vi "VisionGlobal.vi"() -> ()   [LabVIEW 2023]
uses:
  <vilib>/Rock Robotics/WPI/ThirdParty/JAS_Junk/TrajLib/TypeDef/POSE2D.ctl
  <vilib>/Rock Robotics/WPI/ThirdParty/JAS_Junk/TrajLib/TypeDef/TRANSLATION2D.ctl
  <vilib>/Rock Robotics/WPI/ThirdParty/JAS_Junk/TrajLib/TypeDef/ROTATION2D.ctl
  <vilib>/Rock Robotics/WPI/ThirdParty/JAS_Junk/TrajLib/Trajectory_Library.lvlib
panel:
  out "Vision_Right_HasTarg":bool
  out "Vision_Right_NewData":bool
  out "Vision_Left_HasTarg":bool
  out "Vision_Left_NewData":bool
  out "Vision_LeftTime_Sec":dbl
  out "Vision_RightAng_Deg":dbl
  out "Vision_RightY_Ft":dbl
  out "Vision_RightX_Ft":dbl
  out "Vision_RightTime_Sec":dbl
  out "Vision_LeftAng_Deg":dbl
  out "Vision_LeftY_Ft":dbl
  out "Vision_LeftX_Ft":dbl
  out "VisionFPGATime":dbl
  out "Vision Conn L":bool
  out "Vision Count L":dbl=-1.0
  out "Vision Err L":bool
  out "Vision Conn R":bool
  out "Vision Count R":dbl=-1.0
  out "Vision Err R":bool
  out "Odom Error":bool
  in  "Current ABS Pose":T1={"TRANSLATION"={"X"=0.0, "Y"=0.0}, "ROTATION"={"VALUE"=0.0, "COS"=1.0, "SIN"=0.0}} {"ROTATION"."SIN" format="%13.4f"; "ROTATION"."COS" format="%13.4f"; "ROTATION"."VALUE" format="%13.4f"; "TRANSLATION"."Y" format="%14.3f"; "TRANSLATION"."X" format="%14.3f"}
  in  "Initial ABS Pose":T1={"TRANSLATION"={"X"=0.0, "Y"=0.0}, "ROTATION"={"VALUE"=0.0, "COS"=1.0, "SIN"=0.0}} {"ROTATION"."SIN" format="%13.4f"; "ROTATION"."COS" format="%13.4f"; "ROTATION"."VALUE" format="%13.4f"; "TRANSLATION"."Y" format="%14.3f"; "TRANSLATION"."X" format="%14.3f"}
  # "VISION LEFT"
  # "VISION RIGHT"
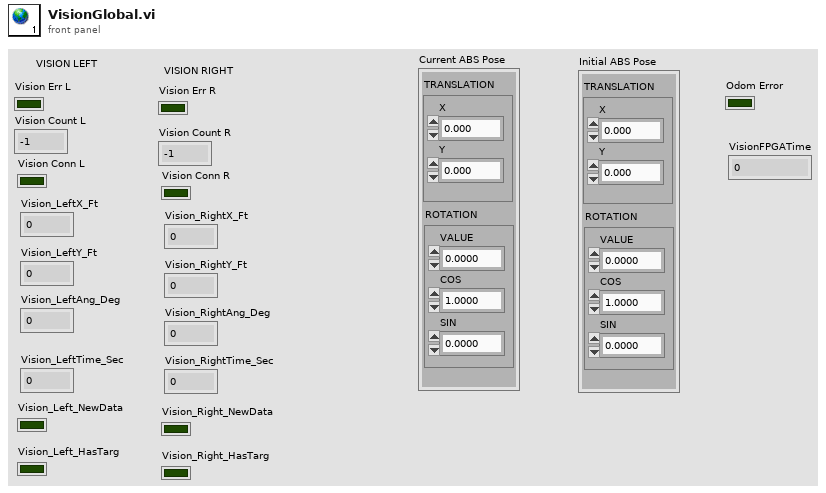
[diagram p1: front panel]
types:
  T1 = typedef "Trajectory_Library.lvlib/POSE2D.ctl" = cluster{"TRANSLATION":T2, "ROTATION":T3}
  T2 = typedef "Trajectory_Library.lvlib/TRANSLATION2D.ctl" = cluster{"X":dbl, "Y":dbl}
  T3 = typedef "Trajectory_Library.lvlib/ROTATION2D.ctl" = cluster{"VALUE":dbl, "COS":dbl, "SIN":dbl}
diagram:
